vi "Lvi Simultaneous Start.vi"(8 "error in (no error)":errorcluster, 10 "NumTasks":u32, 11 "TaskRef":i32[](array[numeric])=array[4097 elements]) -> (0 "error out":errorcluster, 3 "function return":u32(ring))   [LabVIEW 2022 SP3, in "DtLvLink.lvlib"]
doc: "Calls directly into the entry points of the DLL of the Data Acq SDK to explicitly start multiple tasks simultaneously. This VI is used by the higher-level VI, DtOLStart - Simultaneous Start."
uses:
  DtLvLink.lvlib
  <userlib>/LV-Link3/DtLvLink_64.dll
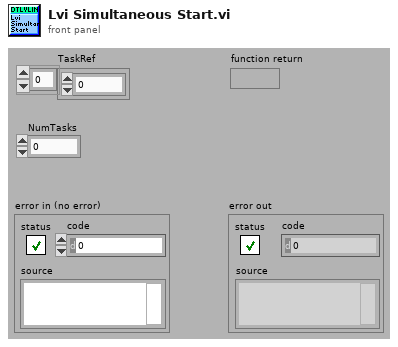
[diagram p1: front panel]
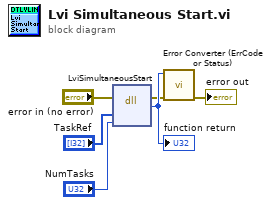
[diagram p0: block diagram]
diagram:
  n1 = dll-call lib="C:/Program Files/National Instruments/LabVIEW 2022/user.lib/LV-Link3/DtLvLink_64.*" fn="LviSimultaneousStart"(error in="error in (no error)", "TaskRef"="TaskRef", "NumTasks"="NumTasks") -> (error out=w2:errorcluster, "return type"=w6:u32)  [unwired: 4 in, 1 out]
  "function return" <- w6
  n2 = call "Error Converter (ErrCode or Status).vi"("error in (no error)"=w2, "error code"=w6) -> ("error out"=→"error out":errorcluster)  [unwired: 9 in]
